vi "encodeArrayInt16.vi"(7 "Compress? (T)":bool=TRUE, 8 "error in (no error)":errorcluster, 11 "Int16 Array":i16[](array[numeric])) -> (0 "error out":errorcluster, 3 "MessagePack":u8[](array[numeric]) format="%.0x")   [LabVIEW 2015, in "MsgPack.lvlib"]
uses:
  MsgPack.lvlib
  encodeInt16.vi
  encodeInt8.vi
  SubVis/encodeFixedInt.vi
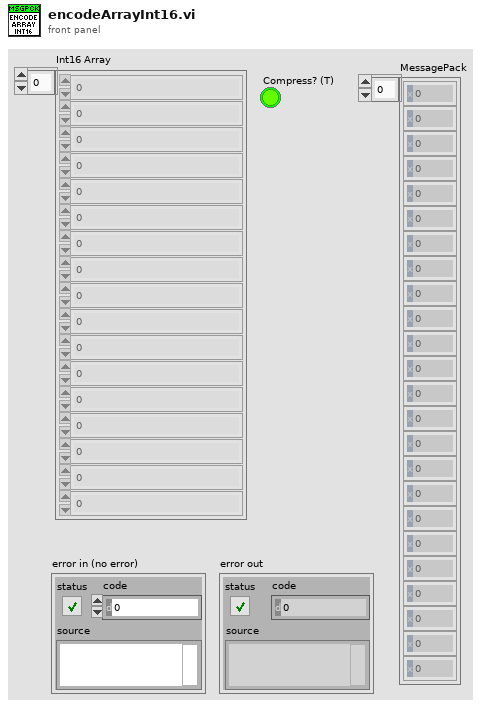
[diagram p1: front panel]
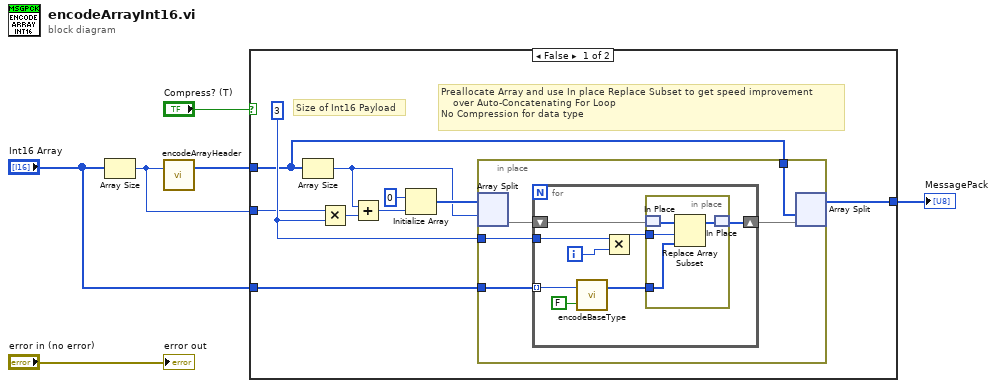
[diagram p0: block diagram]
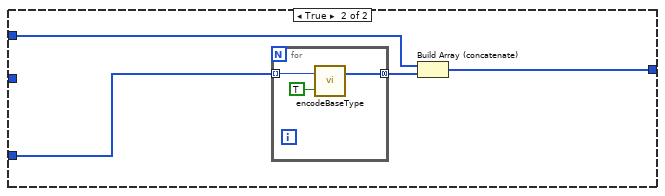
[diagram p2: hidden frame]
diagram:
  n1 = Array Size(array="Int16 Array") -> (size(s)=w5:i32)
  n2 = call "encodeArrayHeader.vi"("Number of Elements"=w5) -> ("array header"=w3:u8[])  [unwired: 2 in]
  n3 = case shown="False" "Compress? (T)" {
    tunnel: [w10 w34] -> w6
    tunnel: w5 -> [w9 _]
    tunnel: "Int16 Array" -> [w8 w35]
    tunnel: w3 -> [w7 w36]
    frame False {
      w11 = 3 ("y")
      # "Preallocate Array and use In place Replace Subset to get speed improvement\n    over Auto-Concatenating For Loop\nNo Compression for data type"
      # "Size of Int16 Payload"
      n4 = Array Size(array=w7) -> (size(s)=w12:i32)
      n5 = Multiply(x=w9, y=w11) -> (x*y=w15:i32)
      n6 = Add(x=w12, y=w15) -> (x+y=w14:i32)
      n7 = Initialize Array(u8 0, w14) -> (w13:u8[])
      n8 = in-place {
        in-place-border: w7 -> [w21]
        in-place-border: w8 -> [w20]
        in-place-border: w11 -> [w17]
        n9 = in-place-split #1(w13, w12) -> (w19:u8[])  [unwired: 1 out]
        n10 = for {
          tunnel: w20 -> [w24] mode=indexing
          shift-right: [w28] -> w18
          shift-left: w19 -> [w29]
          tunnel: w17 -> [w26]
          i -> [w27]
          n11 = call-poly "encodeBaseType.vi"("Compress? (T)"=FALSE ("Compress"), "Int16"=w24) -> ("MessagePack"=w23:u8[])  [unwired: 1 in]
          n12 = Multiply(x=w26, y=w27) -> (x*y=w25:i32)
          n13 = in-place {
            in-place-border: w23 -> [w31]
            in-place-border: w25 -> [w30]
            n14 = in-place-match #2(w29) -> (w33:u8[])
            n15 = Replace Array Subset(array=w33, new element=w31, index=w30) -> (w32:u8[])
            n16 = in-place-match #2(w32) -> (w28:u8[])
          }
        }
        n17 = in-place-split #1(w21, w18) -> (w10:u8[])  [unwired: 1 out]
      }
    }
    frame True {
      n18 = for {
        tunnel: w35 -> [w40] mode=indexing
        tunnel: [w39] -> w37 mode=concatenating
        n19 = call-poly "encodeBaseType.vi"("Compress? (T)"=TRUE ("Compress"), "Int16"=w40) -> ("MessagePack"=w39:u8[])  [unwired: 1 in]
      }
      n20 = Build Array (concatenate)(w36, w37) -> (w34:u8[])
    }
  }
  "MessagePack" <- w6
  "error out" <- "error in (no error)"
